vi "Controller - Timer FGV.vi"(8 "error in (no error)":errorcluster, 10 "Target Time. s":dbl, 11 "Timer CMD":T1) -> (0 "error out":errorcluster, 2 "Elapsed?":bool, 3 "Elapsed Time":dbl)   [LabVIEW 2017]
doc: "FGV Timer for Elevator Controller"
uses:
  Controls/Timer Commands.ctl
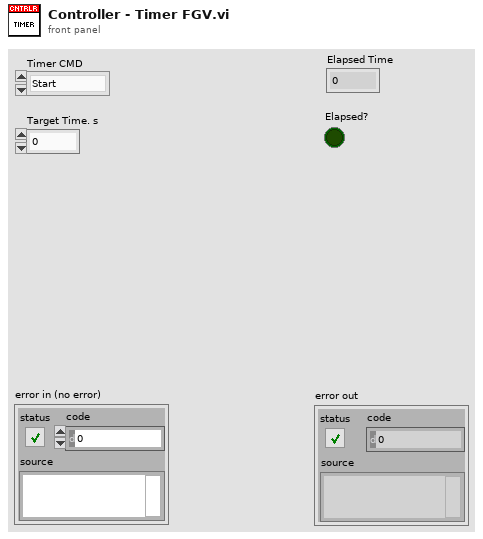
[diagram p1: front panel]
types:
  T1 = typedef "Timer Commands.ctl" = enum16{"Start", "Restart", "Get", "Pause"}
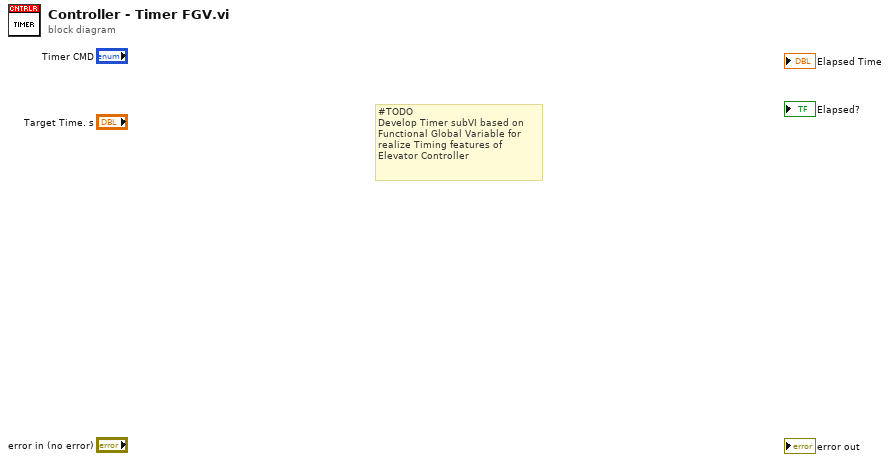
[diagram p0: block diagram]
diagram:
  # "#TODO\nDevelop Timer subVI based on \nFunctional Global Variable for\nrealize Timing features of \nElevator Controller"
